vi "BuildTree.vi"(9 "TreeControl in":refnum<vi>, 10 "Array":T1[](array[typedef])) -> (3 "Map out":map{string, T1}(c390))   [LabVIEW 2024, in "ModuleManager.lvclass"]
uses:
  ModuleManager.lvclass
  RQMHCore/DebugTrace/DebugTraceHandle/StartArgs.ctl
  RQMHCore/DebugTrace/DebugTraceHandle/DebugTraceHandle.lvclass
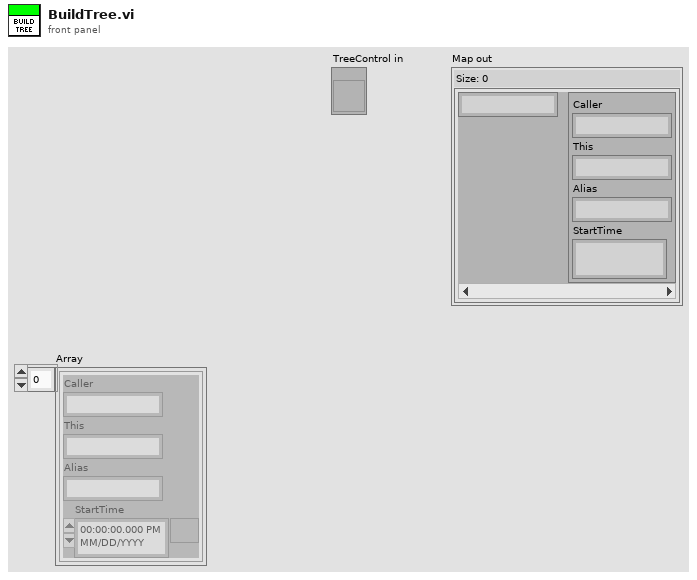
[diagram p1: front panel]
types:
  T1 = typedef "DebugTraceHandle.lvclass/StartArgs.ctl" = cluster{"Caller":string, "This":string, "Alias":string, "StartTime":timestamp}
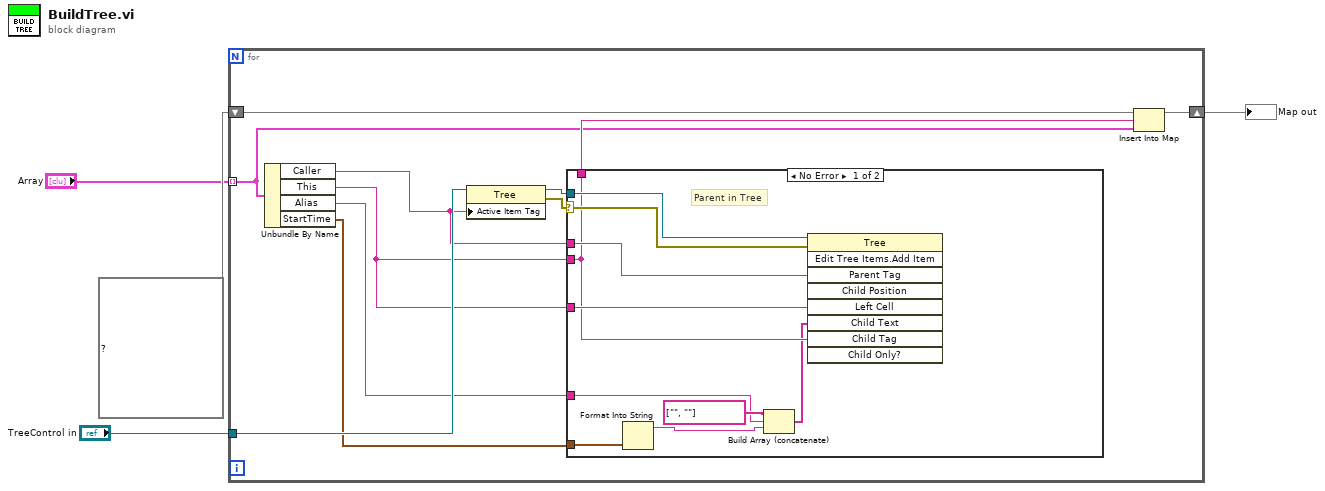
[diagram p0: block diagram]
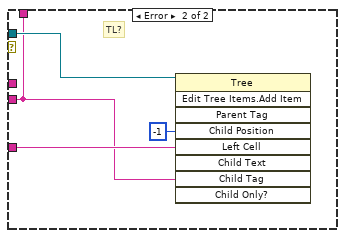
[diagram p2: hidden frame]
diagram:
  n1 = for {
    tunnel: "Array" -> [w7] mode=indexing
    tunnel: "TreeControl in" -> [w15]
    shift-right: [w9] -> w3
    shift-left: map{string, T1} {} ("Map in") -> [w10]
    n2 = Unbundle By Name(w7) -> ("Caller"=w14:string, "This"=w11:string, "Alias"=w6:string, "StartTime"=w5:timestamp)
    n3 = property class="Tree"(reference=w15, "Active Item Tag"=w14) -> (reference out=w12:refnum<vi>, error out=w13:errorcluster)  [unwired: 1 in]
    n4 = case shown="No Error" w13 {
      selector: w13 -> [w24 _]
      tunnel: w12 -> [w25 w29]
      tunnel: w11 -> [w21 w26]
      tunnel: w11 -> [w22 w28]
      tunnel: w14 -> [w23 _]
      tunnel: [w21 w26] -> w8
      tunnel: w6 -> [w18 _]
      tunnel: w5 -> [w17 _]
      frame No Error {
        # "Parent in Tree"
        n5 = Format Into String(w17) -> (resulting string=w16:string)  [unwired: 3 in, 1 out]
        n6 = Build Array (concatenate)(string[] ["", ""], w18, w16) -> (w20:string[])
        n7 = invoke class="Tree" method="Edit Tree Items.Add Item"(reference=w25, error in=w24, "Parent Tag"=w23, "Left Cell"=w22, "Child Text"=w20, "Child Tag"=w21) -> ()  [unwired: 3 in, 9 out]
      }
      frame Error {
        # "TL?"
        n8 = invoke class="Tree" method="Edit Tree Items.Add Item"(reference=w29, "Child Position"=-1, "Left Cell"=w28, "Child Tag"=w26) -> ()  [unwired: 5 in, 9 out]
      }
    }
    n9 = Insert Into Map(map in=w10, key=w8, value=w7) -> (map out=w9:map{string, T1})  [unwired: 2 out]
  }
  "Map out" <- w3
